vi "find_main_contour.vi"(0 "max area":dbl, 10 "contours":T1(array[cluster]), 11 "Y Resolution":i32) -> (1 "max corner":dbl[][](array[numeric]), 2 "Y":dbl[](array[numeric]), 3 "X":dbl[](array[numeric]), 4 "max length ratio":dbl)   [LabVIEW 2017]
panel:
  out "size(s)":i32
  in  "max index":dbl
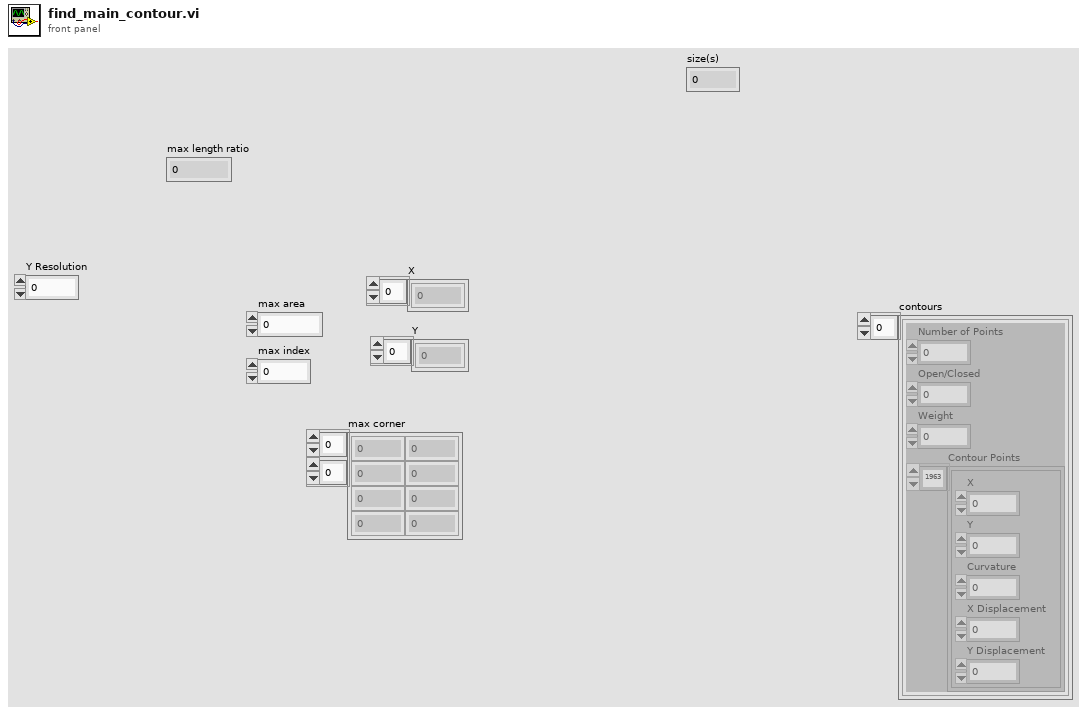
[diagram p1: front panel]
types:
  T1 = cluster{"Number of Points":i32, "Open/Closed":i32, "Weight":dbl, "Contour Points":cluster{"X":dbl, "Y":dbl, "Curvature":dbl, "X Displacement":dbl, "Y Displacement":dbl}[]}[]
  T2 = cluster{"X":dbl, "Y":dbl, "Curvature":dbl, "X Displacement":dbl, "Y Displacement":dbl}[]
  T3 = cluster{"Number of Points":i32, "Open/Closed":i32, "Weight":dbl, "Contour Points":cluster{"X":dbl, "Y":dbl, "Curvature":dbl, "X Displacement":dbl, "Y Displacement":dbl}[]}
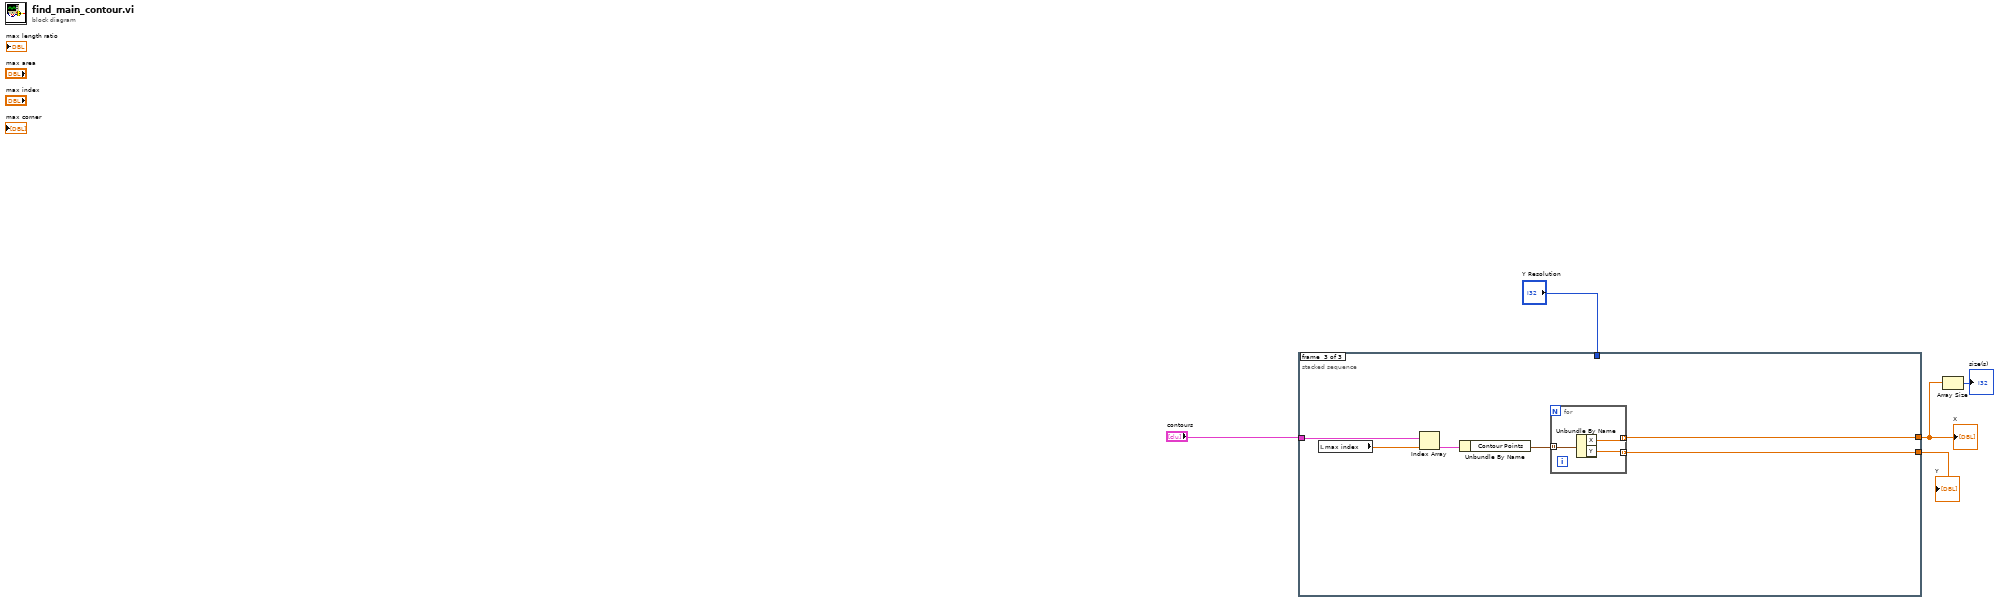
[diagram p0: block diagram]
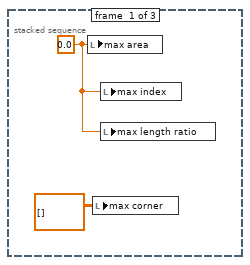
[diagram p2: hidden frame]
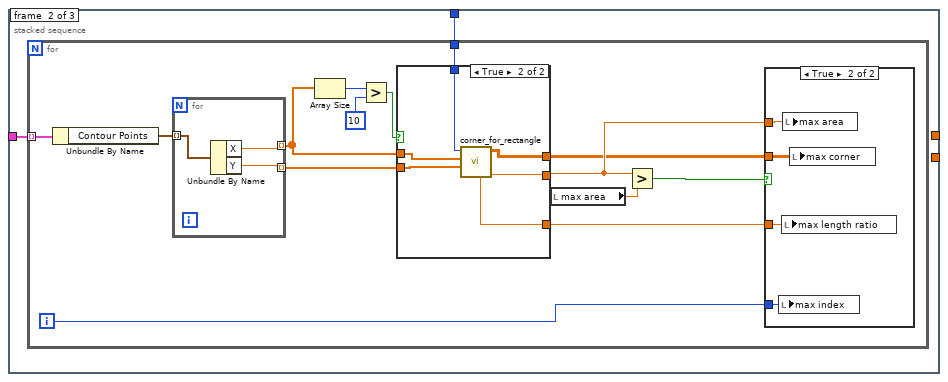
[diagram p3: hidden frame]
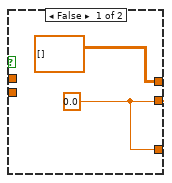
[diagram p5: hidden frame]
diagram:
  n1 = stacked-sequence {
    tunnel: "Y Resolution" -> [_ w9 _]
    tunnel: "contours" -> [_ w8 w44]
    tunnel: [_ _ w41] -> w2
    tunnel: [_ _ w40] -> w4
    frame #0 {
      w6 = 0.0
      n2 = local write "max area"(w6) -> ()
      n3 = local write "max corner"(dbl[][] [] ("max corner")) -> ()
      n4 = local write "max index"(w6) -> ()
      n5 = local write "max length ratio"(w6) -> ()
    }
    frame #1 {
      n6 = for {
        tunnel: w8 -> [w23] mode=indexing
        tunnel: w9 -> [w16]
        i -> [w12]
        n7 = Unbundle By Name(w23) -> ("Contour Points"=w22:T2)
        n8 = for {
          tunnel: w22 -> [w38] mode=indexing
          tunnel: [w37] -> w18 mode=indexing
          tunnel: [w36] -> w17 mode=indexing
          n9 = Unbundle By Name(w38) -> ("X"=w37:dbl, "Y"=w36:dbl)
        }
        n10 = Array Size(array=w18) -> (size(s)=w21:i32)
        n11 = Greater?(x=w21, y=10) -> (0:w19:bool)
        n12 = case shown="True" w19 {
          tunnel: w18 -> [_ w35]
          tunnel: w17 -> [_ w34]
          tunnel: w16 -> [_ w33]
          tunnel: [w28 w32] -> w13
          tunnel: [dbl[][] [] ("max corner") w31] -> w11
          tunnel: [w28 w30] -> w10
          frame False {
            w28 = 0.0
          }
          frame True {
            n13 = call "corner_for_rectangle.vi"("Y"=w34, "X"=w35, "Y Resolution"=w33) -> ("area"=w32:dbl, "corner"=w31:dbl[][], "length ratio"=w30:dbl)  [unwired: 6 in]
          }
        }
        n14 = local read "max area"() -> (w15:dbl)
        n15 = Greater?(x=w13, y=w15) -> (0:w14:bool)
        n16 = case shown="True" w14 {
          tunnel: w13 -> [_ w27]
          tunnel: w12 -> [_ w26]
          tunnel: w11 -> [_ w25]
          tunnel: w10 -> [_ w24]
          frame False {
          }
          frame True {
            n17 = local write "max index"(w26) -> ()
            n18 = local write "max length ratio"(w24) -> ()
            n19 = local write "max area"(w27) -> ()
            n20 = local write "max corner"(w25) -> ()
          }
        }
      }
    }
    frame #2 {
      n21 = local read "max index"() -> (w39:dbl)
      n22 = Index Array(array=w44, index=w39) -> (element=w43:T3)
      n23 = Unbundle By Name(w43) -> ("Contour Points"=w42:T2)
      n24 = for {
        tunnel: w42 -> [w47] mode=indexing
        tunnel: [w46] -> w41 mode=indexing
        tunnel: [w45] -> w40 mode=indexing
        n25 = Unbundle By Name(w47) -> ("X"=w46:dbl, "Y"=w45:dbl)
      }
    }
  }
  "X" <- w2
  "Y" <- w4
  n26 = Array Size(array=w2) -> (size(s)=→"size(s)":i32)
